vi "StartSequenceAcqusition.vi"(0 "Camera_Prime95B in":refnum<class "Camera_Prime95B.lvclass">, 5 "Exposure":i32=100, 7 "BufferSize":i32=100, 9 "SavingPath":string="C:\\temp.tiff", 11 "error in (no error)":errorcluster) -> (4 "Camera_Prime95B out":refnum<class "Camera_Prime95B.lvclass">, 15 "error out":errorcluster)   [LabVIEW 2020, in "Camera_Prime95B.lvlib" / "Camera_Prime95B.lvclass"]
uses:
  Camera_Prime95B.lvclass
  Camera_Prime95B.lvclass/Camera_Prime95B.ctl
  E:/Development/DevHardSoftware/MMicroscopyAF/Model/Real Hardware/Camera_Prime95B/Camera_Prime95B/Dependencies/PVCamNET.dll
  Dependencies/PVCamNET.dll
  Camera New Frame Arrived Callback.vi
  HAL Layer/Camera/Camera/Camera.lvclass
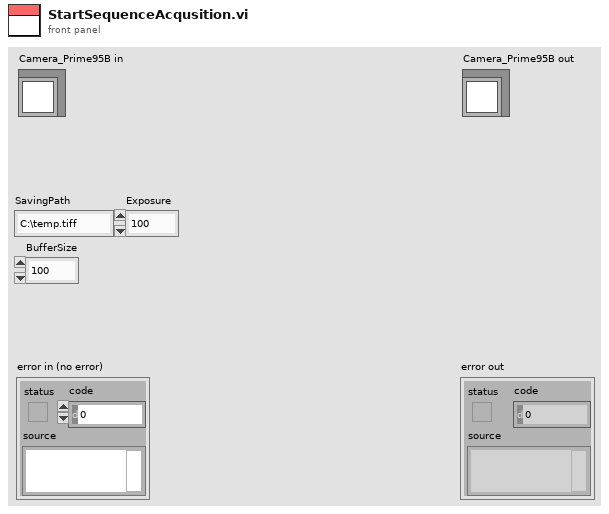
[diagram p1: front panel]
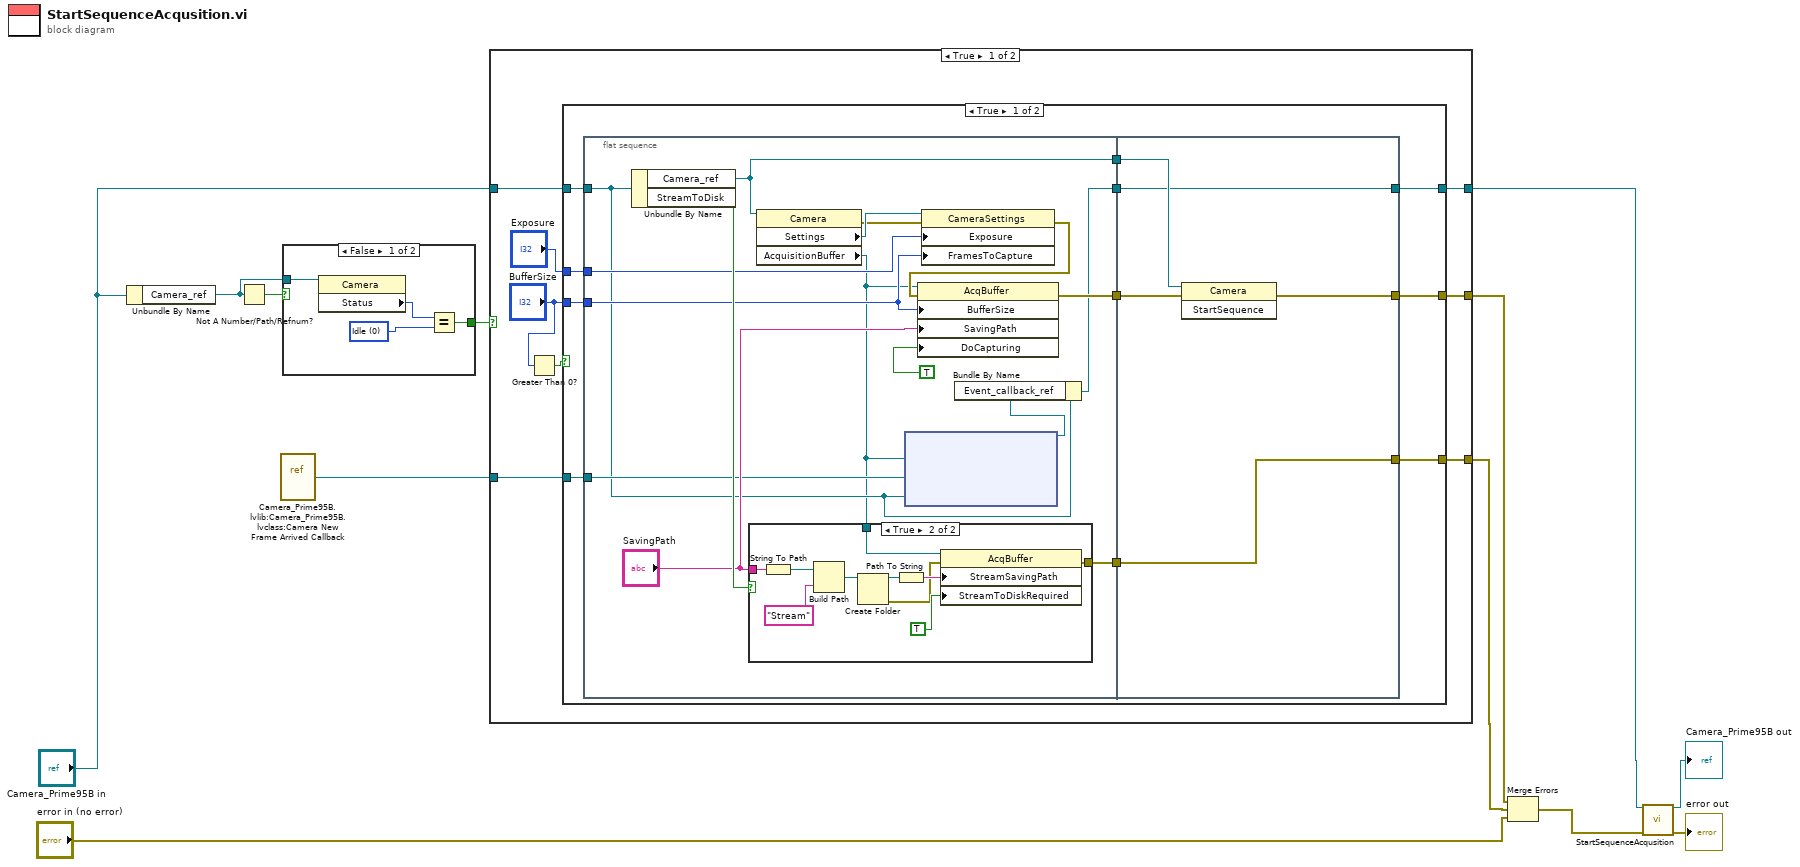
[diagram p0: block diagram]
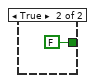
[diagram p2: hidden frame]
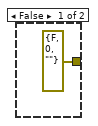
[diagram p3: hidden frame]
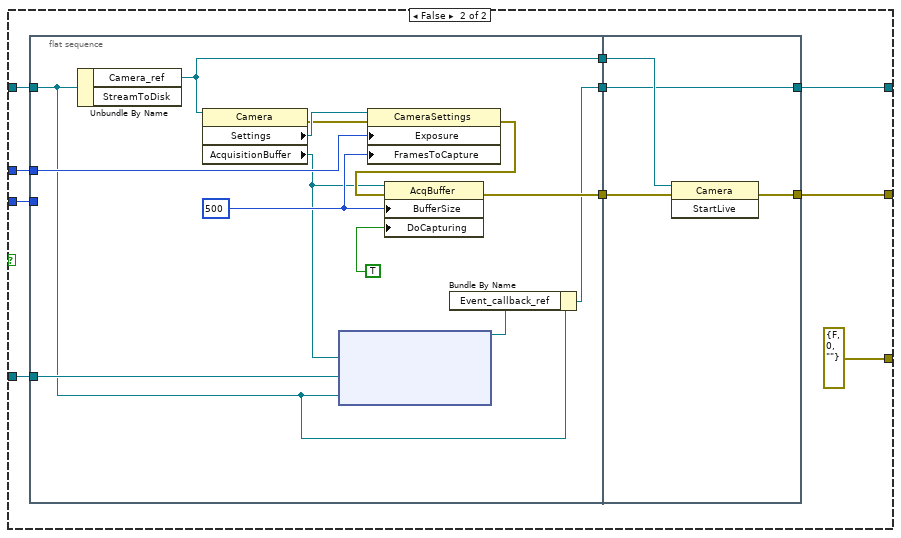
[diagram p4: hidden frame]
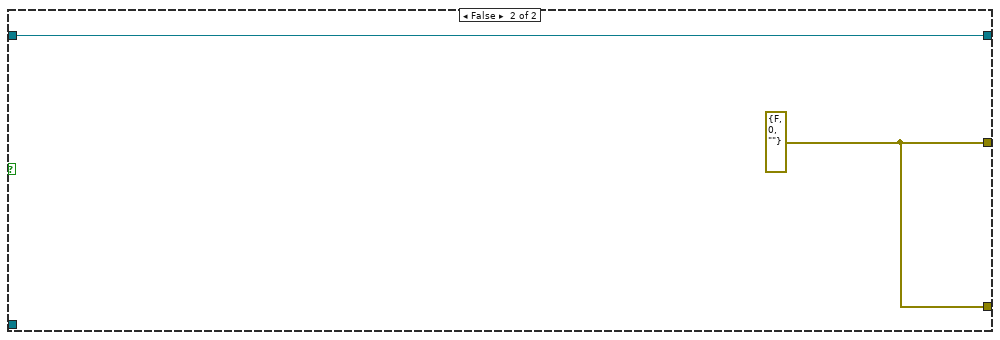
[diagram p5: hidden frame]
diagram:
  n1 = Unbundle By Name("Camera_Prime95B in") -> ("Camera_ref"=w10:refnum<k24>)
  n2 = Not A Number/Path/Refnum?(number/path/refnum=w10) -> (NaN/Path/Refnum?=w12:bool)
  n3 = vi-ref "Camera_Prime95B.lvlib:Camera_Prime95B.lvclass:Camera New Frame Arrived Callback.vi"() -> ("vi reference"=w3:refnum<vi>)
  n4 = case shown="False" w12 {
    tunnel: [w14 FALSE] -> w11
    tunnel: w10 -> [w13 _]
    frame False {
      w16 = 0 items=["Idle", "Capturing"] ("Status")
      n5 = property class="Camera"(reference=w13) -> ("Status"=w15:i32)  [unwired: 1 in, 2 out]
      n6 = Equal?(x=w15, y=w16) -> (x = y?=w14:bool)
    }
    frame True {
    }
  }
  n7 = case shown="True" w11 {
    tunnel: "Camera_Prime95B in" -> [w25 w96]
    tunnel: [w24 w97] -> w8
    tunnel: [w23 w97] -> w4
    tunnel: w3 -> [w19 _]
    tunnel: [w18 w96] -> w1
    frame True {
      n8 = Greater Than 0?(x="BufferSize") -> (x > 0?=w21:bool)
      n9 = case shown="True" w21 {
        tunnel: w25 -> [w33 w76]
        tunnel: [w32 w75] -> w24
        tunnel: [w31 errorcluster {"status"=FALSE, "code"=0, "source"=""} ("error out")] -> w23
        tunnel: "BufferSize" -> [w30 w74]
        tunnel: "Exposure" -> [w29 w73]
        tunnel: w19 -> [w28 w71]
        tunnel: [w26 w70] -> w18
        frame True {
          n10 = flat-sequence {
            tunnel: w33 -> [w40]
            tunnel: [w49] -> w36
            tunnel: [w48] -> w35
            tunnel: [w44] -> w34
            tunnel: w30 -> [w43]
            tunnel: w29 -> [w42]
            tunnel: w28 -> [w41]
            tunnel: [w38] -> w27
            tunnel: w36 -> [w68]
            tunnel: w35 -> [w67]
            tunnel: [w66] -> w32
            tunnel: [w65] -> w31
            tunnel: w34 -> [w65]
            tunnel: [w64] -> w26
            tunnel: w27 -> [w64]
            frame #0 {
              n11 = Unbundle By Name(w40) -> ("Camera_ref"=w49:refnum<k24>, "StreamToDisk"=w46:bool)
              n12 = property class="Camera"(reference=w49) -> (error out=w51:errorcluster, "Settings"=w52:refnum<k24>, "AcquisitionBuffer"=w37:refnum<k24>)  [unwired: 1 in, 1 out]
              n13 = case shown="True" w46 {
                tunnel: "SavingPath" -> [_ w62]
                tunnel: w37 -> [_ w56]
                tunnel: [errorcluster {"status"=FALSE, "code"=0, "source"=""} ("error out") w54] -> w44
                frame False {
                }
                frame True {
                  n14 = String To Path(string=w62) -> (path=w63:path)
                  n15 = Build Path(base path=w63, name or relative path="Stream") -> (appended path=w60:path)
                  n16 = Create Folder(path (use dialog)=w60) -> (created path=w59:path, error out=w55:errorcluster)  [unwired: 2 in, 1 out]
                  n17 = Path To String(path=w59) -> (string=w57:string)
                  n18 = property class="AcqBuffer"(reference=w56, error in=w55, "StreamSavingPath"=w57, "StreamToDiskRequired"=TRUE) -> (error out=w54:errorcluster)  [unwired: 1 out]
                }
              }
              n19 = node(w37, w41, w40) -> (w39:refnum<k27>)  [unwired: 2 in, 1 out]
              n20 = property class="CameraSettings"(reference=w52, error in=w51, "Exposure"=w42, "FramesToCapture"=w43) -> (error out=w50:errorcluster)  [unwired: 1 out]
              n21 = property class="AcqBuffer"(reference=w37, error in=w50, "BufferSize"=w43, "SavingPath"="SavingPath", "DoCapturing"=TRUE) -> (error out=w48:errorcluster)  [unwired: 1 out]
              n22 = Bundle By Name(cluster=w40, "Event_callback_ref"=w39) -> (w38:refnum<class "Camera_Prime95B.lvclass">)
            }
            frame #1 {
              n23 = invoke class="Camera" method="StartSequence"(reference=w68, error in=w67) -> (error out=w66:errorcluster)  [unwired: 1 in, 2 out]
            }
          }
        }
        frame False {
          n24 = flat-sequence {
            tunnel: w76 -> [w81]
            tunnel: [w88] -> w78
            tunnel: [w87] -> w77
            tunnel: w74 -> [_]
            tunnel: w73 -> [w85]
            tunnel: w71 -> [w82]
            tunnel: [w79] -> w69
            tunnel: w78 -> [w95]
            tunnel: w77 -> [w94]
            tunnel: [w93] -> w75
            tunnel: [w92] -> w70
            tunnel: w69 -> [w92]
            frame #0 {
              w84 = u16 500 ("FramesToCapture")
              n25 = Unbundle By Name(w81) -> ("Camera_ref"=w88:refnum<k24>)  [unwired: 1 out]
              n26 = property class="Camera"(reference=w88) -> (error out=w90:errorcluster, "Settings"=w91:refnum<k24>, "AcquisitionBuffer"=w83:refnum<k24>)  [unwired: 1 in, 1 out]
              n27 = node(w83, w82, w81) -> (w80:refnum<k27>)  [unwired: 2 in, 1 out]
              n28 = property class="CameraSettings"(reference=w91, error in=w90, "Exposure"=w85, "FramesToCapture"=w84) -> (error out=w89:errorcluster)  [unwired: 1 out]
              n29 = property class="AcqBuffer"(reference=w83, error in=w89, "BufferSize"=w84, "DoCapturing"=TRUE) -> (error out=w87:errorcluster)  [unwired: 1 out]
              n30 = Bundle By Name(cluster=w81, "Event_callback_ref"=w80) -> (w79:refnum<class "Camera_Prime95B.lvclass">)
            }
            frame #1 {
              n31 = invoke class="Camera" method="StartLive"(reference=w95, error in=w94) -> (error out=w93:errorcluster)  [unwired: 1 in, 2 out]
            }
          }
        }
      }
    }
    frame False {
      w97 = errorcluster {"status"=FALSE, "code"=0, "source"=""} ("error out")
    }
  }
  n32 = Merge Errors(w8, w4, "error in (no error)") -> (w6:errorcluster)
  n33 = call-parent "StartSequenceAcqusition.vi"("Camera in"=w1, "error in (no error)"=w6) -> ("Camera out"=→"Camera_Prime95B out":refnum<class "Camera_Prime95B.lvclass">, "error out"=→"error out":errorcluster)  [unwired: 12 in]
